vi "write pulse test.vi"   [LabVIEW 2015]
types:
  T1 = enum16{"init", "config", "start", "write", "stop"}
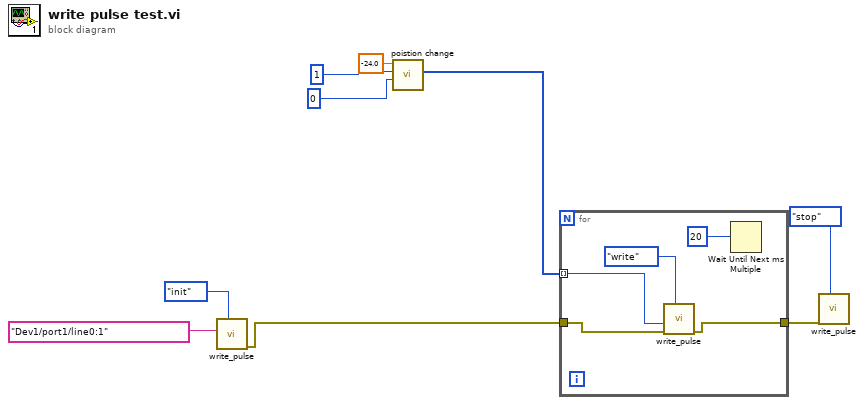
[diagram p0: block diagram]
diagram:
  n1 = call "write_pulse.vi"("Enum"=T1."init", "lines"=tag "Dev1/port1/line0:1") -> ("error out"=w1:errorcluster)  [unwired: 8 in]
  n2 = call "poistion change.vi"("Value"=-24.0, "方向"=u32 1, "位置"=u32 0) -> ("Data"=w2:u8[])  [unwired: 6 in]
  n3 = for {
    tunnel: w2 -> [w11] mode=indexing
    tunnel: w1 -> [w13]
    tunnel: [w12] -> w7
    n4 = call "write_pulse.vi"("Enum"=T1."write", "error in"=w13, "data"=w11) -> ("error out"=w12:errorcluster)  [unwired: 7 in]
    n5 = Wait Until Next ms Multiple(millisecond multiple=u32 20) -> ()  [unwired: 1 out]
  }
  n6 = call "write_pulse.vi"("Enum"=T1."stop", "error in"=w7) -> ()  [unwired: 8 in, 1 out]
